vi "Write.vi"(8 "error in (no error)":errorcluster, 9 "timeout ms (25000)":i32, 10 "Bytes to write":u8[](array[numeric]), 11 "VISA TCP in":refnum<class "VISA TCP.lvclass">) -> (0 "error out":errorcluster, 1 "timed out?":bool, 2 "bytes written":i32, 3 "VISA TCP out":refnum<class "VISA TCP.lvclass">)   [LabVIEW 2021, in "Sockets.lvlib" / "VISA TCP.lvclass"]
doc: "Writes data to the socket.\nWebSockets 2.0.1.40\nSam Sharp - MediaMongrels Ltd\nCopyright (c) 2019, MediaMongrels Ltd"
uses:
  VISA TCP.lvclass
  VISA TCP.lvclass/VISA TCP.ctl
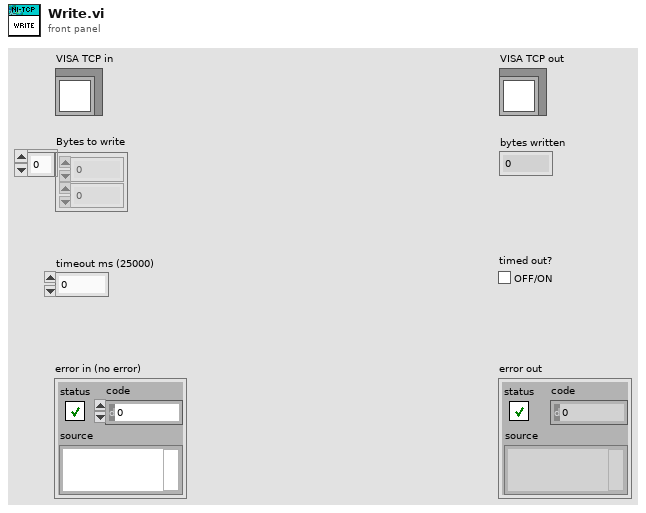
[diagram p1: front panel]
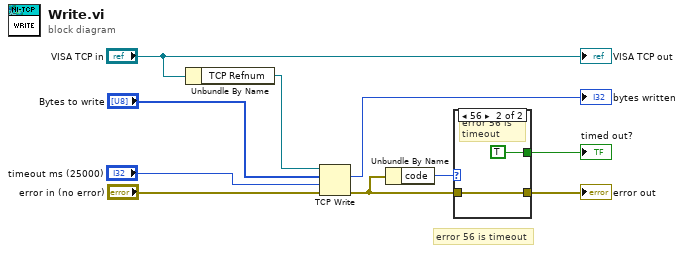
[diagram p0: block diagram]
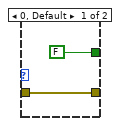
[diagram p2: hidden frame]
diagram:
  # "error 56 is timeout"
  n1 = Unbundle By Name("VISA TCP in") -> ("TCP Refnum"=w8:refnum<k5>)
  n2 = TCP Write(connection ID=w8, data in="Bytes to write", error in (no error)="error in (no error)", 9:"timeout ms (25000)") -> (bytes written=→"bytes written":i32, error out=w10:errorcluster)  [unwired: 1 out]
  n3 = Unbundle By Name(w10) -> ("code"=w9:i32)
  n4 = case shown="56" w9 {
    tunnel: w10 -> [w12 w13]
    tunnel: [w12 w13] -> w5
    tunnel: [FALSE TRUE] -> w1
    frame 0, Default {
    }
    frame 56 {
      # "error 56 is timeout"
    }
  }
  "error out" <- w5
  "timed out?" <- w1
  "VISA TCP out" <- "VISA TCP in"
